vi "VI Tree.vi"   [LabVIEW 2013, in "Agilent 3446X Series.lvlib"]
doc: "This is the instrument driver for the Agilent 3446X Series. The VI Tree displays all the user-callable VIs of the instrument driver in an organized table."
uses:
  Agilent 3446X Series.lvlib
  Data/Read (Single Point).vi
panel:
  # "(c) 2013 National Instruments.  ALL RIGHTS RESERVED."
  # "SEE DIAGRAM\nFOR VI TREE."
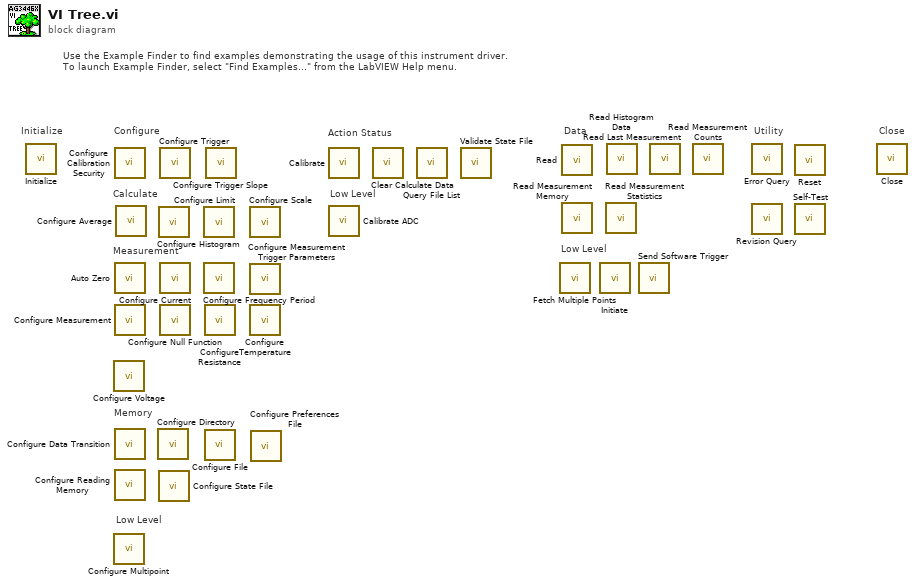
[diagram p0: block diagram]
diagram:
  # "Memory"
  # "Measurement"
  # "Calculate"
  # "Low Level"
  # "Action Status"
  # "Low Level"
  # "Low Level"
  # "Use the Example Finder to find examples demonstrating the usage of this instrument driver.\nTo launch Example Finder, select \"Find Examples...\" from the LabVIEW Help menu."
  # "Configure"
  # "Utility"
  # "Data"
  # "Close"
  # "Initialize"
  n1 = call "Initialize.vi"() -> ()  [unwired: 10 in, 2 out]
  n2 = call "Configure Voltage.vi"() -> ()  [unwired: 10 in, 2 out]
  n3 = call "Configure Multipoint.vi"() -> ()  [unwired: 10 in, 2 out]
  n4 = call "Configure Calibration Security.vi"() -> ()  [unwired: 10 in, 2 out]
  n5 = call "Auto Zero.vi"() -> ()  [unwired: 10 in, 2 out]
  n6 = call "Configure Measurement.vi"() -> ()  [unwired: 10 in, 2 out]
  n7 = call "Configure Data Transition.vi"() -> ()  [unwired: 10 in, 2 out]
  n8 = call "Configure Reading Memory.vi"() -> ()  [unwired: 10 in, 2 out]
  n9 = call "Configure Average.vi"() -> ()  [unwired: 10 in, 2 out]
  n10 = call "Configure Directory.vi"() -> ()  [unwired: 10 in, 2 out]
  n11 = call "Configure Histogram.vi"() -> ()  [unwired: 10 in, 2 out]
  n12 = call "Configure State File.vi"() -> ()  [unwired: 10 in, 2 out]
  n13 = call "Configure Trigger.vi"() -> ()  [unwired: 10 in, 2 out]
  n14 = call "Configure Current.vi"() -> ()  [unwired: 10 in, 2 out]
  n15 = call "Configure Null Function.vi"() -> ()  [unwired: 10 in, 2 out]
  n16 = call "Configure Limit.vi"() -> ()  [unwired: 10 in, 2 out]
  n17 = call "Configure Frequency Period.vi"() -> ()  [unwired: 10 in, 2 out]
  n18 = call "Configure Resistance.vi"() -> ()  [unwired: 10 in, 2 out]
  n19 = call "Configure File.vi"() -> ()  [unwired: 10 in, 2 out]
  n20 = call "Configure Trigger Slope.vi"() -> ()  [unwired: 10 in, 2 out]
  n21 = call "Configure Scale.vi"() -> ()  [unwired: 10 in, 2 out]
  n22 = call "Configure Measurement Trigger Parameters.vi"() -> ()  [unwired: 10 in, 2 out]
  n23 = call "Configure Temperature.vi"() -> ()  [unwired: 10 in, 2 out]
  n24 = call "Configure Preferences File.vi"() -> ()  [unwired: 10 in, 2 out]
  n25 = call "Calibrate.vi"() -> ()  [unwired: 9 in, 3 out]
  n26 = call "Calibrate ADC.vi"() -> ()  [unwired: 9 in, 3 out]
  n27 = call "Clear Calculate Data.vi"() -> ()  [unwired: 10 in, 2 out]
  n28 = call "Query File List.vi"() -> ()  [unwired: 7 in, 5 out]
  n29 = call "Validate State File.vi"() -> ()  [unwired: 9 in, 3 out]
  n30 = call "Fetch Multiple Points.vi"() -> ()  [unwired: 9 in, 3 out]
  n31 = call-poly "Read.vi"() -> ()  [unwired: 9 in, 3 out]
  n32 = call "Read Measurement Memory .vi"() -> ()  [unwired: 9 in, 3 out]
  n33 = call "Initiate.vi"() -> ()  [unwired: 10 in, 2 out]
  n34 = call "Read Measurement Statistics.vi"() -> ()  [unwired: 8 in, 8 out]
  n35 = call "Read Histogram Data.vi"() -> ()  [unwired: 9 in, 3 out]
  n36 = call "Send Software Trigger.vi"() -> ()  [unwired: 10 in, 2 out]
  n37 = call "Read Last Measurement.vi"() -> ()  [unwired: 9 in, 3 out]
  n38 = call "Read Measurement Counts.vi"() -> ()  [unwired: 9 in, 3 out]
  n39 = call "Error Query.vi"() -> ()  [unwired: 8 in, 4 out]
  n40 = call "Revision Query.vi"() -> ()  [unwired: 8 in, 4 out]
  n41 = call "Reset.vi"() -> ()  [unwired: 10 in, 2 out]
  n42 = call "Self-Test.vi"() -> ()  [unwired: 8 in, 4 out]
  n43 = call "Close.vi"() -> ()  [unwired: 11 in, 1 out]
